vi "ERR HANDLER - Trap Error.vi"(8 "error in":errorcluster) -> ()   [LabVIEW 2013]
uses:
  Error Queue Message.ctl
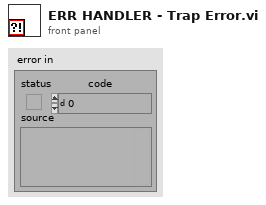
[diagram p1: front panel]
types:
  T1 = typedef "Error Queue Message.ctl" = cluster{"Command":enum16{"HANDLE ERROR", "EXIT"}, "Data":variant}
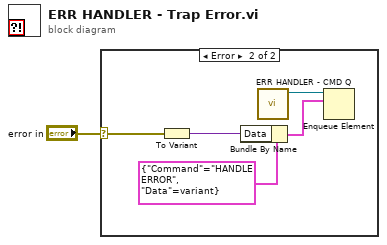
[diagram p0: block diagram]
diagram:
  n1 = case shown="Error" "error in" {
    selector: "error in" -> [_ w5]
    frame No Error {
    }
    frame Error {
      n2 = To Variant(anything=w5) -> (Variant=w6:variant)
      n3 = Bundle By Name(cluster=T1 {"Command"=enum."HANDLE ERROR", "Data"=variant} ("Error Handler Mesg"), "Data"=w6) -> (w2:T1)
      n4 = call "ERR HANDLER - CMD Q.vi"() -> ("Err Handler Q"=w3:refnum<queue>)  [unwired: 11 in]
      n5 = Enqueue Element(queue=w3, element=w2) -> ()  [unwired: 2 in, 3 out]
    }
  }
